vi "Pre-Build VI - Run Unit Tests.vi"(8 "error in (no error)":errorcluster, 11 "Fail on #todo items":bool) -> (0 "error out":errorcluster, 1 "VIs without test coverage":string[](array[string]), 2 "error type":enum16{"fatal", "non-fatal", "warning"}(ring), 3 "num tests":i32, 4 "VIs not loadable":string[](array[string]), 5 "VIs Failed":string[](array[string]), 6 "VIs with #todo bookmarks":string[](array[string]))   [LabVIEW 2020]
uses:
  <vilib>/Utility/miscctls.llb/LVBookmarkInfoTypeDef.ctl
  <vilib>/addons/_JKI Toolkits/Caraya/run-tests/Run Test (Scalar Path).vi
  <vilib>/addons/_JKI Toolkits/Caraya/Caraya.lvlib
panel:
  out "VIs with #todo's":map{path, T1}(c390)
  out "VIs Succeeded":string[](array[string])
  in  "type specifier VI Refnum (for type only)":refnum<vi>
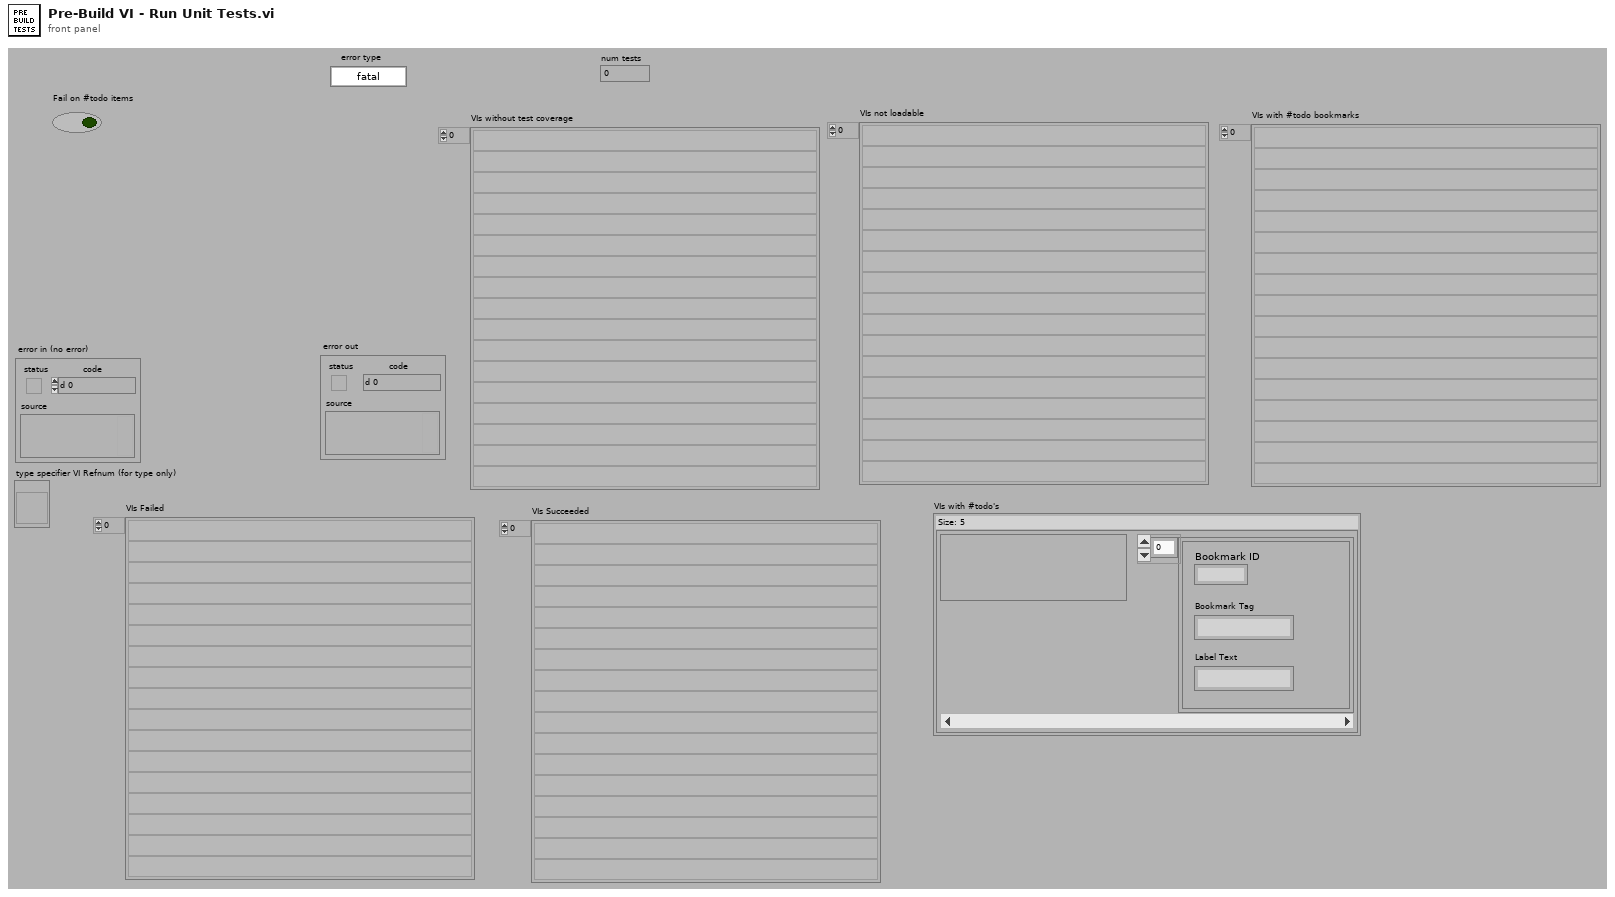
[diagram p1: front panel]
types:
  T1 = typedef "LVBookmarkInfoTypeDef.ctl" = cluster{"Bookmark ID":u32, "Bookmark Tag":string, "Label Text":string}[]
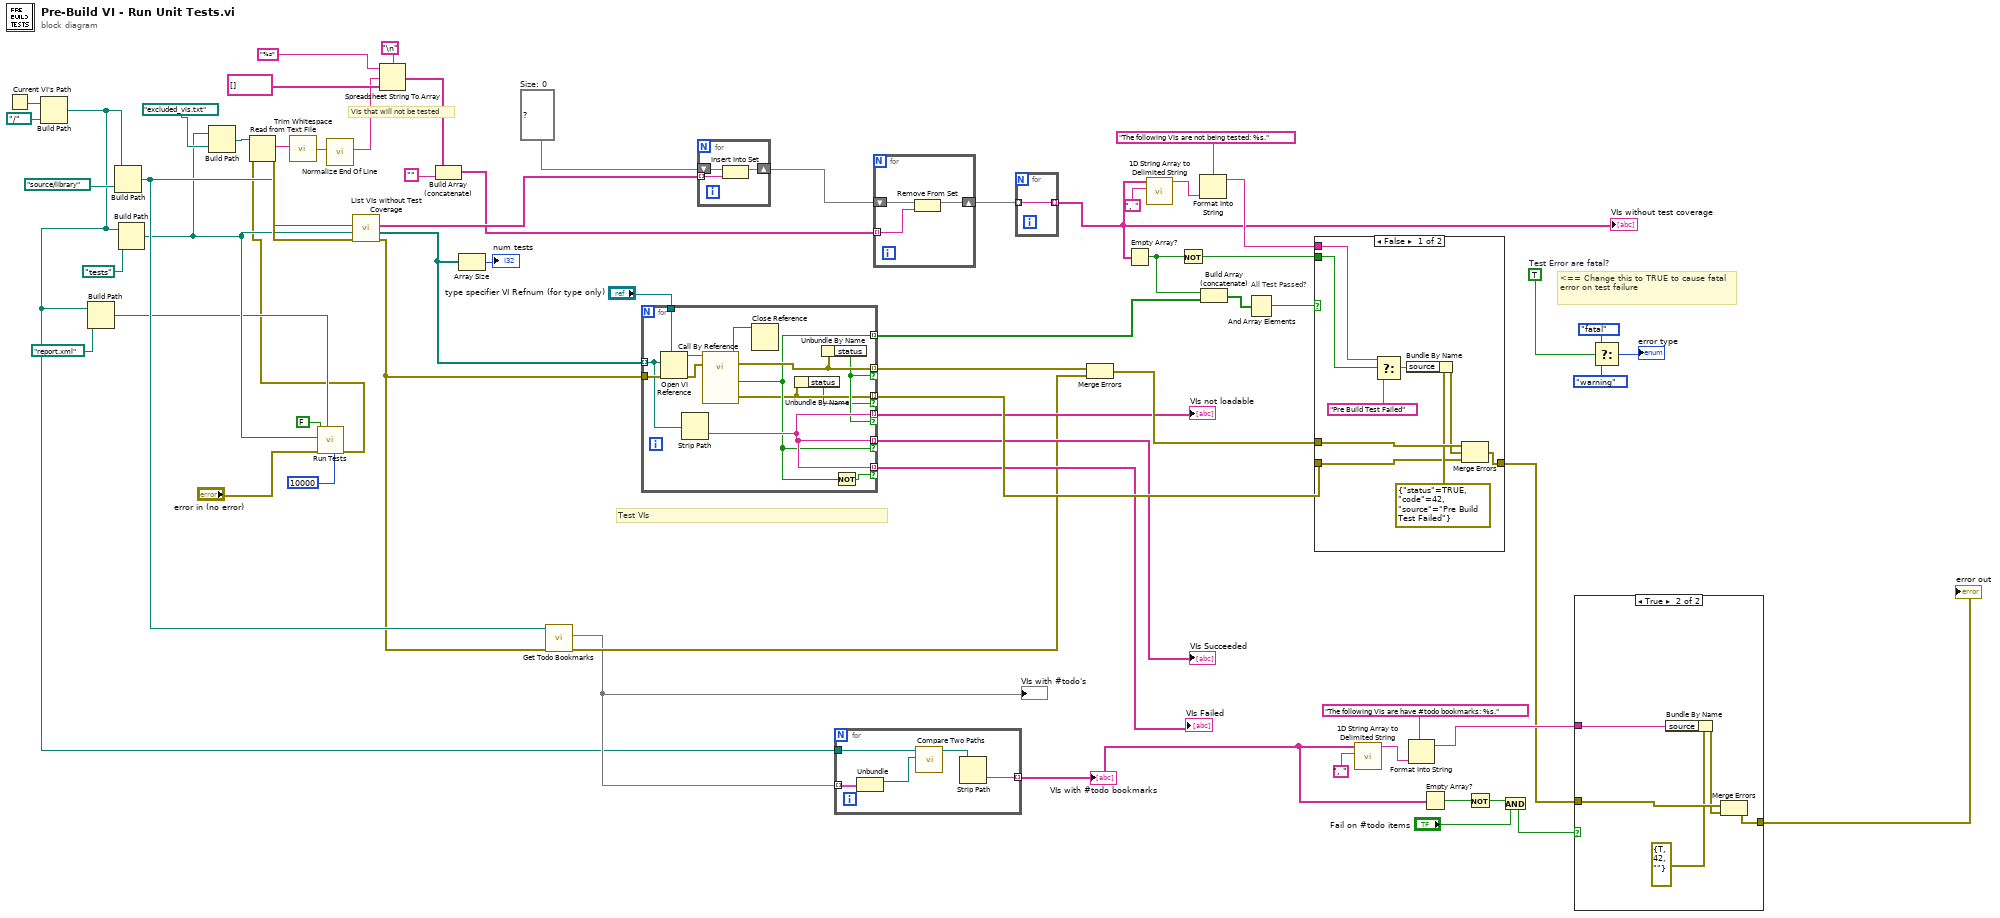
[diagram p0: block diagram]
diagram:
  w40 = set{string} {}  # Size: 0
  w59 = TRUE  # Test Error are fatal?
  # "VIs that will not be tested"
  # "<== Change this to TRUE to cause fatal error on test failure"
  # "All Test Passed?"
  # "Test VIs"
  n1 = Current VI's Path() -> (path=w46:path)
  n2 = Build Path(base path=w46, name or relative path=path "../..") -> (appended path=w7:path)
  n3 = Build Path(base path=w7, name or relative path=path "report.xml" ("Relative path (.)")) -> (appended path=w5:path)
  n4 = Build Path(base path=w7, name or relative path=path "source/library" ("Relative path (.)")) -> (appended path=w24:path)
  n5 = Build Path(base path=w7, name or relative path=path "tests" ("Relative path (.)")) -> (appended path=w9:path)
  n6 = Build Path(base path=w9, name or relative path=path "excluded_vis.txt" ("Relative path (.)")) -> (appended path=w41:path)
  n7 = call-poly <vilib>:"Run Tests.vi"("timeout (2000 ms)"=10000, "Report Path"=w5, "error in"="error in (no error)", "Test Path"=w9, "Interactive (T)"=FALSE) -> ("error out"=w2:errorcluster)  [unwired: 5 in, 1 out]
  n8 = Read from Text File(file (use dialog)=w41, error in=w2) -> (text=w28:string, error out=w27:errorcluster)  [unwired: 2 in, 2 out]
  n9 = call <vilib>:"Trim Whitespace.vi"("string"=w28) -> ("trimmed string"=w30:string)  [unwired: 1 in]
  n10 = call <vilib>:"Normalize End Of Line.vi"("string in"=w30) -> ("string out"=w29:string)  [unwired: 7 in]
  n11 = call "List VIs without Test Coverage.vi"("error in (no error)"=w27, "Tests Root"=w9, "Source Root"=w24) -> ("error out"=w21:errorcluster, "Test VIs"=w26:path[], "VIs without test coverage"=w39:string[])  [unwired: 6 in]
  n12 = Spreadsheet String To Array(delimiter (Tab)="\n", format string="%s", spreadsheet string=w29, array type (2D Dbl)=string[] [] ("appended array")) -> (array=w31:string[])
  n13 = Build Array (concatenate)(w31, "") -> (w37:string[])
  n14 = Array Size(array=w26) -> (size(s)=→"num tests":i32)
  n15 = call "Get Todo Bookmarks.vi"("error in (no error)"=w21, "Directory to Search"=w24) -> ("error out"=w23:errorcluster, "todo bookmarks"=w13:map{path, T1})  [unwired: 8 in]
  "VIs with #todo's" <- w13
  n16 = for {
    tunnel: w26 -> [w73] mode=indexing
    tunnel: "type specifier VI Refnum (for type only)" -> [w79]
    tunnel: [w71] -> w50 mode=indexing
    tunnel: [w68] -> w54 mode=indexing if=w67
    tunnel: w21 -> [w75]
    tunnel: [w74] -> w51 mode=indexing if=w69
    tunnel: [w72] -> w49 mode=indexing if=w69
    tunnel: [w72] -> w48 mode=indexing if=w71
    tunnel: [w72] -> w47 mode=indexing if=w70
    n17 = Open VI Reference(type specifier VI Refnum (for type only)=w79, vi path=w73, error in (no error)=w75) -> (vi reference=w78:refnum<vi>, error out=w77:errorcluster)  [unwired: 3 in]
    n18 = Strip Path(path=w73) -> (name=w72:string)  [unwired: 1 out]
    n19 = call-by-ref "?"(reference=w78, error in=w77) -> (reference out=w76:refnum<vi>, error out=w74:errorcluster, 0:"error out"=w68:errorcluster, "pass"=w71:bool)  [unwired: 10 in]
    n20 = Close Reference(reference=w76) -> ()  [unwired: 1 in, 1 out]
    n21 = Unbundle By Name(w68) -> ("status"=w67:bool)
    n22 = Unbundle By Name(w74) -> ("status"=w69:bool)
    n23 = Not(x=w71) -> (.not. x?=w70:bool)
  }
  "VIs not loadable" <- w49
  "VIs Succeeded" <- w48
  "VIs Failed" <- w47
  n24 = for {
    tunnel: w39 -> [w82] mode=indexing
    shift-right: [w80] -> w38
    shift-left: w40 -> [w81]
    n25 = Insert Into Set(10:w82, 11:w81) -> (3:w80:set{string})  [unwired: 1 out]
  }
  n26 = for {
    tunnel: w13 -> [w87] mode=indexing
    tunnel: w7 -> [w85]
    tunnel: [w83] -> w16 mode=indexing
    n27 = Unbundle(w87) -> ("key type"=w86:path)  [unwired: 1 out]
    n28 = call <vilib>:"Compare Two Paths.vi"("Path 2"=w86, "Path 1"=w85) -> ("Relative Path from 1 to 2"=w84:path)  [unwired: 6 in, 3 out]
    n29 = Strip Path(path=w84) -> (name=w83:string)  [unwired: 1 out]
  }
  "VIs with #todo bookmarks" <- w16
  n30 = for {
    shift-right: [w88] -> w36
    shift-left: w38 -> [w90]
    tunnel: w37 -> [w89] mode=indexing
    n31 = Remove From Set(10:w89, 11:w90) -> (3:w88:set{string})  [unwired: 1 out]
  }
  n32 = for {
    tunnel: [w91] -> w35 mode=indexing
    tunnel: w36 -> [w91] mode=indexing
  }
  "VIs without test coverage" <- w35
  n33 = Merge Errors(w51, w23) -> (w52:errorcluster)
  n34 = Empty Array?(array=w35) -> (empty?=w61:bool)
  n35 = call <vilib>:"1D String Array to Delimited String.vi"("delimiter"=", " ("delimiter (Tab)"), "string array"=w35) -> ("delimited string"=w64:string)  [unwired: 9 in]
  n36 = Not(x=w61) -> (.not. x?=w60:bool)
  n37 = Format Into String(format string="The following VIs are not being tested: %s.", w64) -> (resulting string=w62:string)  [unwired: 2 in, 1 out]
  n38 = Build Array (concatenate)(w61, w50) -> (w22:bool[])
  n39 = And Array Elements(Boolean array=w22) -> (logical AND=w66:bool)
  n40 = case shown="False" w66 {
    tunnel: w52 -> [w100 w101]
    tunnel: [w99 w101] -> w14
    tunnel: w60 -> [w98 _]
    tunnel: w62 -> [w97 _]
    tunnel: w54 -> [w92 _]
    frame False {
      n41 = Select(t=w97, s=w98, f="Pre Build Test Failed" ("source")) -> (s? t:f=w95:string)
      n42 = Bundle By Name(cluster=errorcluster {"status"=TRUE, "code"=42, "source"="Pre Build Test Failed"} ("error out"), "source"=w95) -> (w94:errorcluster)
      n43 = Merge Errors(w100, w94, w92) -> (w99:errorcluster)
    }
    frame True {
    }
  }
  n44 = call <vilib>:"1D String Array to Delimited String.vi"("delimiter"=", " ("delimiter (Tab)"), "string array"=w16) -> ("delimited string"=w19:string)  [unwired: 9 in]
  n45 = Format Into String(format string="The following VIs are have #todo bookmarks: %s.", w19) -> (resulting string=w17:string)  [unwired: 2 in, 1 out]
  n46 = Empty Array?(array=w16) -> (empty?=w15:bool)
  n47 = Not(x=w15) -> (.not. x?=w12:bool)
  n48 = And(x=w12, y="Fail on #todo items") -> (x .and. y?=w11:bool)
  n49 = case shown="True" w11 {
    tunnel: w14 -> [w102 w107]
    tunnel: [w102 w103] -> w1
    tunnel: w17 -> [_ w104]
    frame False {
    }
    frame True {
      n50 = Bundle By Name(cluster=errorcluster {"status"=TRUE, "code"=42, "source"=""} ("error out"), "source"=w104) -> (w106:errorcluster)
      n51 = Merge Errors(w107, w106) -> (w103:errorcluster)
    }
  }
  "error out" <- w1
  n52 = Select(t=enum16{"fatal", "non-fatal", "warning"}."fatal" ("error type"), s=w59, f=enum16{"fatal", "non-fatal", "warning"}."warning" ("error type")) -> (s? t:f=→"error type":enum16{"fatal", "non-fatal", "warning"})
